vi "IDSinit.vi"(7 "error in (no error)":errorcluster, 10 "Camera ID":i32) -> (0 "error out":errorcluster, 1 "Cam Info":T1, 2 "Ranges":T3, 3 "reference out":refnum<k24>)   [LabVIEW 2018]
uses:
  <vilib>/Utility/miscctls.llb/LVMinMaxIncTypeDef.ctl
  C:/Program Files/National Instruments/LabVIEW 2018/instr.lib/IDS/ueye.NET/uEyeDotNet.dll
  instr.lib/IDS/ueye.NET/uEyeDotNet.dll
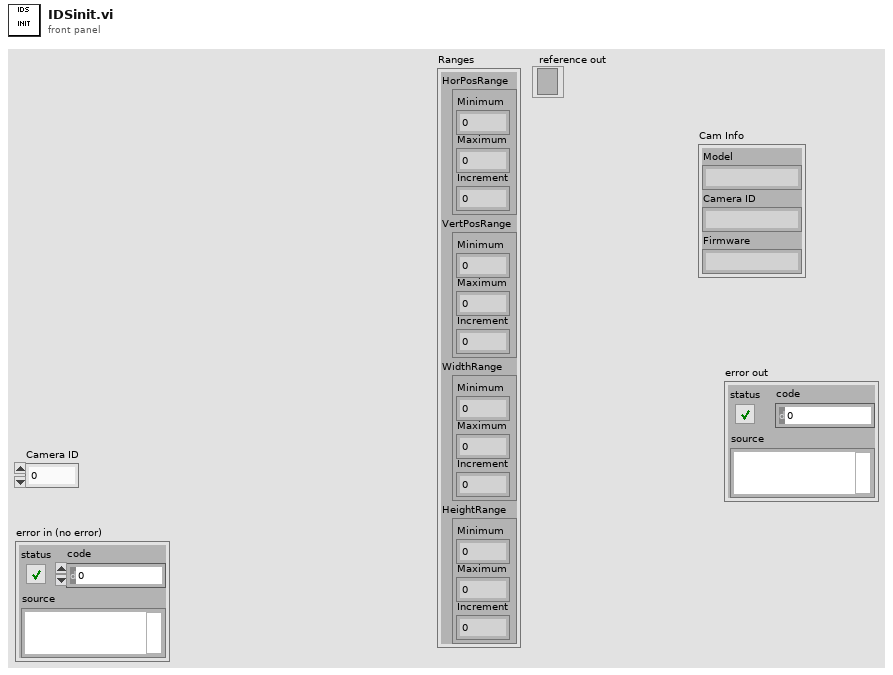
[diagram p1: front panel]
types:
  T1 = cluster{"Model":string, "Camera ID":string, "Firmware":string}
  T2 = typedef "LVMinMaxIncTypeDef.ctl" = cluster{"Minimum":dbl, "Maximum":dbl, "Increment":dbl}
  T3 = cluster{"HorPosRange":T2, "VertPosRange":T2, "WidthRange":T2, "HeightRange":T2}
  T4 = cluster{"Data Entry Limits":T2, "Data Entry Limits":T2, "Data Entry Limits":T2, "Data Entry Limits":T2}
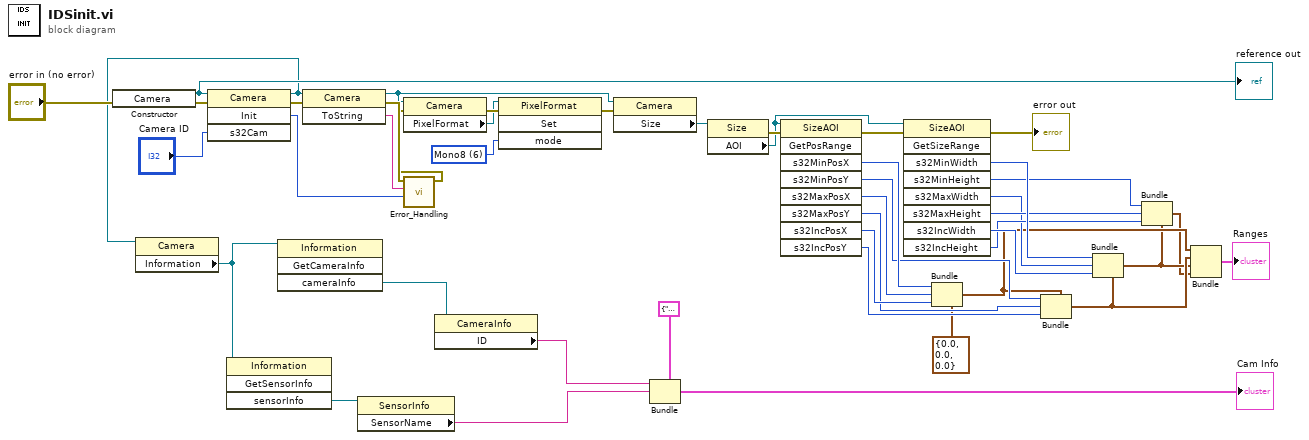
[diagram p0: block diagram]
diagram:
  w11 = 6 items=["BGRA8Packed"=0, "BGR8Packed"=1, "BGR565Packed"=2, "BGR5Packed"=3, "Mono8"=6, "SensorRaw8"=11, "UYVYPacked"=12, "UYVYMonoPacked"=13, "UYVYBayerPacked"=14, "CBYCRYPacked"=23, "BGRY8Packed"=24, "BGR10Packed"=25, "Mono12"=26, "SensorRaw12"=27, "Mono16"=28, "SensorRaw16"=29, "BGR12Unpacked"=30, "BGRA12Unpacked"=31, "Jpeg"=32, "BGR10Unpacked"=35, "RGBA8Packed"=128, "RGB8Packed"=129, "RGBY8Packed"=152, "RGB10Packed"=153, "RGB12Unpacked"=158, "RGBA12Unpacked"=159, "RGB10Unpacked"=163, "RGB8Planar"=8321, "PreferPackedSourceFormat"=16384] ("mode")
  n1 = constructor class="Camera"(error in="error in (no error)") -> (reference out=w10:refnum<k24>, error out=w44:errorcluster)  [unwired: 2 in, 1 out]
  "reference out" <- w10
  n2 = invoke class="Camera" method="Init"(reference=w10, error in=w44, "s32Cam"="Camera ID") -> (reference out=w5:refnum<k24>, error out=w42:errorcluster, "Init"=w40:i32)  [unwired: 1 in, 1 out]
  n3 = property class="Camera"(reference=w5) -> ("Information"=w4:refnum<k24>)  [unwired: 1 in, 2 out]
  n4 = invoke class="Information" method="GetSensorInfo"(reference=w4) -> ("sensorInfo"=w3:refnum<k24>)  [unwired: 3 in, 3 out]
  n5 = invoke class="Information" method="GetCameraInfo"(reference=w4) -> ("cameraInfo"=w9:refnum<k24>)  [unwired: 3 in, 3 out]
  n6 = invoke class="Camera" method="ToString"(reference=w5, error in=w42) -> (reference out=w14:refnum<k24>, error out=w39:errorcluster, "ToString"=w41:string)  [unwired: 1 in]
  n7 = property class="SensorInfo"(reference=w3) -> ("SensorName"=w2:string)  [unwired: 1 in, 2 out]
  n8 = call <instrlib>:"Error_Handling.vi"("Error Code"=w40, "Error String"=w41, "Error In"=w39) -> ("Error Out"=w1:errorcluster)  [unwired: 8 in]
  n9 = property class="Camera"(reference=w14, error in=w1) -> (error out=w15:errorcluster, "PixelFormat"=w13:refnum<k24>)  [unwired: 1 out]
  n10 = property class="CameraInfo"(reference=w9) -> ("ID"=w7:string)  [unwired: 1 in, 2 out]
  n11 = invoke class="PixelFormat" method="Set"(reference=w13, error in=w15, "mode"=w11) -> (error out=w12:errorcluster)  [unwired: 1 in, 3 out]
  n12 = property class="Camera"(reference=w14, error in=w12) -> ("Size"=w22:refnum<k24>)  [unwired: 2 out]
  n13 = Bundle(cluster=T1 {"Model"="", "Camera ID"="", "Firmware"=""} ("Camera Details"), "Model"=w7, "Camera ID"=w2) -> (→"Cam Info":T1)  [unwired: 1 in]
  n14 = property class="Size"(reference=w22) -> (error out=w31:errorcluster, "AOI"=w29:refnum<k24>)  [unwired: 1 in, 1 out]
  n15 = invoke class="SizeAOI" method="GetPosRange"(reference=w29, error in=w31) -> (error out=w30:errorcluster, "s32MinPosX"=w38:i32, "s32MinPosY"=w35:i32, "s32MaxPosX"=w37:i32, "s32MaxPosY"=w34:i32, "s32IncPosX"=w36:i32, "s32IncPosY"=w33:i32)  [unwired: 7 in, 2 out]
  n16 = invoke class="SizeAOI" method="GetSizeRange"(reference=w29, error in=w30) -> (error out=→"error out":errorcluster, "s32MinWidth"=w26:i32, "s32MinHeight"=w23:i32, "s32MaxWidth"=w21:i32, "s32MaxHeight"=w25:i32, "s32IncWidth"=w27:i32, "s32IncHeight"=w24:i32)  [unwired: 7 in, 2 out]
  n17 = Bundle(cluster=T2 {"Minimum"=0.0, "Maximum"=0.0, "Increment"=0.0} ("Data Entry Limits"), "Minimum"=w38, "Maximum"=w37, "Increment"=w36) -> (w20:T2)
  n18 = Bundle(cluster=w20, "Minimum"=w35, "Maximum"=w34, "Increment"=w33) -> (w19:T2)
  n19 = Bundle(cluster=w19, "Minimum"=w26, "Maximum"=w21, "Increment"=w27) -> (w18:T2)
  n20 = Bundle(cluster=w18, "Minimum"=w23, "Maximum"=w25, "Increment"=w24) -> (w17:T2)
  n21 = Bundle("Data Entry Limits"=w20, "Data Entry Limits"=w19, "Data Entry Limits"=w18, "Data Entry Limits"=w17) -> (→"Ranges":T4)  [unwired: 1 in]
